vi "Motor Control.vi"(0 "Right Motor":dbl(knob) scale=-100.0..100.0, 1 "Motor Frequency":dbl=2500.0, 2 "Left Motor":dbl(knob) scale=-100.0..100.0) -> ()   [LabVIEW 2013]
uses:
  <vilib>/myRIO/Instrument Drivers/Onboard IO/DIO/vis/Smart Open.vi
  <vilib>/myRIO/Instrument Drivers/Onboard IO/DIO/vis/Write.vi
  <vilib>/myRIO/Instrument Drivers/Onboard IO/PWM/vis/Smart Open.vi
  <vilib>/myRIO/Instrument Drivers/Onboard IO/PWM/vis/Set Duty Cycle and Frequency.vi
  <vilib>/myRIO/Instrument Drivers/Onboard IO/DIO/vis/Open.vi
  <vilib>/myRIO/Instrument Drivers/Onboard IO/PWM/vis/Open.vi
  <vilib>/myRIO/Common/Instrument Driver Framework/myRIO v1.0/DIO/vis/myRIO v1.1 Open DIO.vi
  <vilib>/myRIO/Common/Instrument Driver Framework/myRIO v1.0/PWM/vis/myRIO v1.1 Open PWM.vi
  <vilib>/myRIO/Common/Instrument Driver Framework/Utilities/vis/Validate Channels.vi
  <vilib>/myRIO/Common/Instrument Driver Framework/myRIO v1.0/DIO/vis/myRIO v1.0 Reserve DIO.vi
  <vilib>/myRIO/Common/Instrument Driver Framework/myRIO v1.0/PWM/vis/myRIO v1.0 Reserve PWM.vi
  <vilib>/myRIO/Common/Instrument Driver Framework/myRIO v1.0/Resource Manager/vis/myRIO v1.0 Reserve Channel List.vi
  <vilib>/myRIO/Common/Instrument Driver Framework/myRIO v1.0/DIO/vis/myRIO v1.0 Build MUX Configuration DIO.vi
  <vilib>/myRIO/Common/Instrument Driver Framework/myRIO v1.0/PWM/vis/myRIO v1.0 Build MUX Configuration PWM.vi
  <vilib>/myRIO/Common/Instrument Driver Framework/myRIO v1.0/Resource Manager/vis/myRIO v1.0 Reserve Channel.vi
  <vilib>/myRIO/Common/Instrument Driver Framework/myRIO v1.0/Resource Manager/vis/myRIO v1.0 Unreserve Channel.vi
  <vilib>/myRIO/Common/Instrument Driver Framework/myRIO v1.0/Resource Manager/vis/myRIO v1.0 Create Configuration List.vi
  <vilib>/myRIO/Common/Instrument Driver Framework/myRIO v1.0/Resource Manager/vis/myRIO v1.0 Build Mutex Name.vi
  <vilib>/myRIO/Common/Instrument Driver Framework/myRIO v1.0/myRIO v1.1 Open.vi
  <vilib>/Utility/VariantDataType/GetNumericInfo.vi
  <vilib>/Utility/error.llb/Error Cluster From Error Code.vi
  <vilib>/myRIO/Common/Instrument Driver Framework/Utilities/vis/IO Manager.vi
  <vilib>/myRIO/Common/Instrument Driver Framework/Utilities/vis/Configuration Manager.vi
  <vilib>/myRIO/Common/Instrument Driver Framework/myRIO v1.0/Resource Manager/vis/myRIO v1.0 Configure IO.vi
  <vilib>/myRIO/Common/Instrument Driver Framework/myRIO v1.0/myRIO v1.0 Close.vi
  <vilib>/myRIO/Common/Instrument Driver Framework/myRIO v1.0/DIO/vis/myRIO v1.0 Write DIO.vi
  <vilib>/myRIO/Common/Instrument Driver Framework/myRIO v1.0/PWM/vis/myRIO v1.0 Write PWM.vi
panel:
  # "MOT1A  - LR\nMOT1B  - LG\nMOT2A  - RR\nMOT2B  - RG"
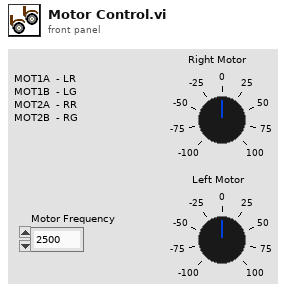
[diagram p1: front panel]
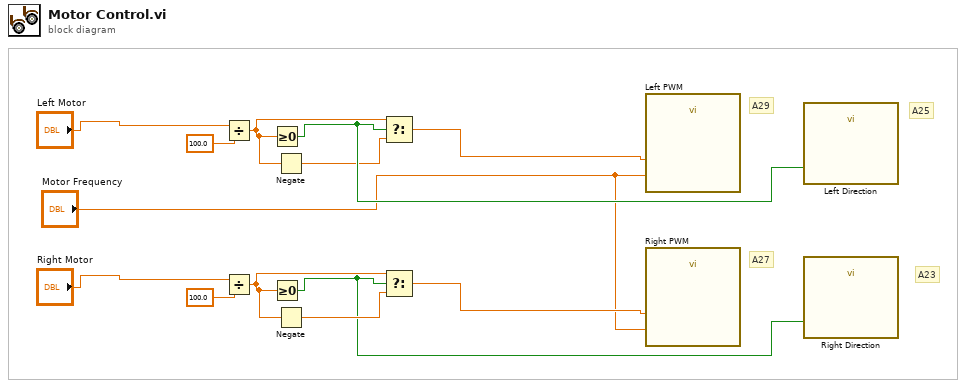
[diagram p0: block diagram]
diagram:
  # "A23"
  # "A25"
  # "A27"
  # "A29"
  n1 = Divide(x="Left Motor", y=100.0) -> (x/y=w9:dbl)
  n2 = Divide(x="Right Motor", y=100.0) -> (x/y=w8:dbl)
  n3 = Greater Or Equal To 0?(x=w9) -> (x >= 0?=w11:bool)
  n4 = Greater Or Equal To 0?(x=w8) -> (x >= 0?=w6:bool)
  n5 = Negate(x=w9) -> (-x=w10:dbl)
  n6 = Negate(x=w8) -> (-x=w7:dbl)
  n7 = Select(t=w9, s=w11, f=w10) -> (s? t:f=w12:dbl)
  n8 = Select(t=w8, s=w6, f=w7) -> (s? t:f=w5:dbl)
  n9 = call "Left PWM"("Duty Cycle (0-1)"=w12, "Frequency (Hz)"="Motor Frequency") -> ()  [unwired: 25 in, 1 out]
  n10 = call "Right PWM"("Duty Cycle (0-1)"=w5, "Frequency (Hz)"="Motor Frequency") -> ()  [unwired: 25 in, 1 out]
  n11 = call "Left Direction"("A/DIO7 (Pin 25)"=w11) -> ()  [unwired: 26 in, 1 out]
  n12 = call "Right Direction"("A/DIO6 (Pin 23)"=w6) -> ()  [unwired: 26 in, 1 out]
